vi "up_grid_data.vi"(9 "Data.V_Downstream":T1, 10 "Data.V_UpStream":T1) -> (0 "DOWN_Angle [Deg]":dbl, 1 "UP_Angle [Deg]":dbl, 2 "upper layer grid info":T3, 5 "DOWN_Angle_unwrap":dbl, 7 "UP_Angle_unwrap":dbl)   [LabVIEW 2021]
uses:
  3ph Phasor.ctl
  Phasor.ctl
  <vilib>/Analysis/coordinate.llb/Wrap Angle (scalar).vi
  <vilib>/Analysis/baseanly.llb/Complex A x Vector.vi
  <vilib>/Analysis/baseanly.llb/Mean (DBL).vi
  <vilib>/Analysis/Matrix/Numeric/Conversions/Array To Matrix - CA2.vi
  <vilib>/Analysis/NI_AALBase.lvlib
  <vilib>/Analysis/Matrix/NI_Matrix.lvlib
  <vilib>/Analysis/NI_AAL_Angle.lvlib
  <vilib>/Analysis/NI_AALPro.lvlib
panel:
  in  "y":dbl
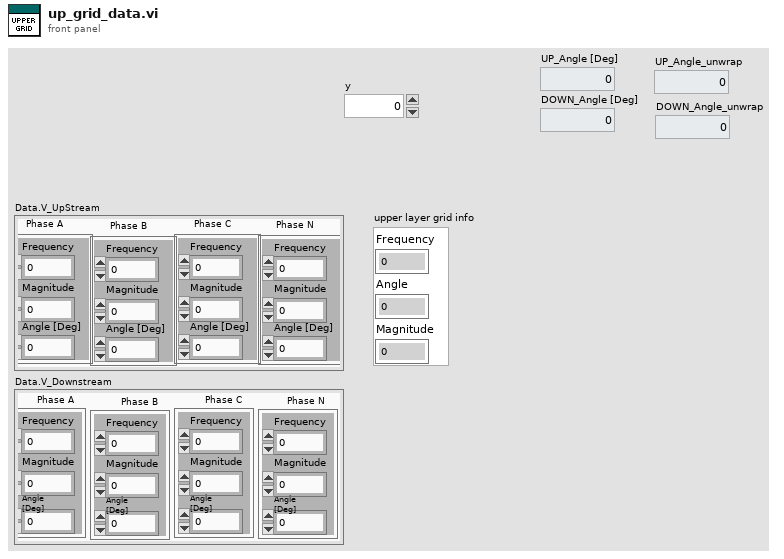
[diagram p1: front panel]
types:
  T1 = typedef "3ph Phasor.ctl" = cluster{"Phase A":T2, "Phase B":T2, "Phase C":T2, "Phase N":T2}
  T2 = typedef "Phasor.ctl" = cluster{"Frequency":dbl, "Magnitude":dbl, "Angle [Deg]":dbl}
  T3 = cluster{"Frequency":dbl, "Angle":dbl, "Magnitude":dbl}
  T4 = typedef "NI_Matrix.lvlib/ComplexMatrix.ctl" = cdb[][]
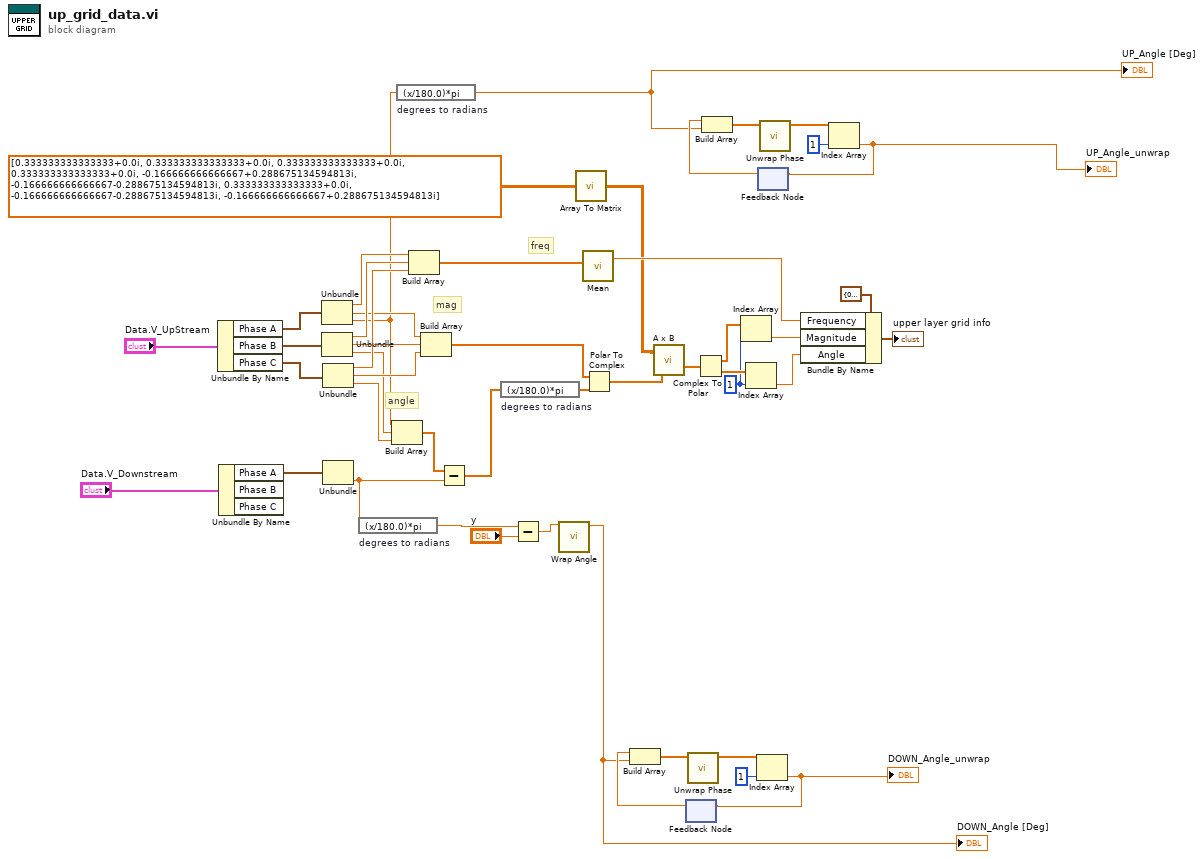
[diagram p0: block diagram]
diagram:
  w27 = 1 ("index")
  # "angle"
  # "mag"
  # "freq"
  n1 = Unbundle By Name("Data.V_UpStream") -> ("Phase A"=w45:T2, "Phase B"=w44:T2, "Phase C"=w43:T2)
  n2 = Unbundle By Name("Data.V_Downstream") -> ("Phase A"=w26:T2)  [unwired: 2 out]
  n3 = Unbundle(w45) -> ("Frequency"=w42:dbl, "Magnitude"=w39:dbl, "Angle [Deg]"=w17:dbl)
  n4 = Unbundle(w44) -> ("Frequency"=w41:dbl, "Magnitude"=w38:dbl, "Angle [Deg]"=w36:dbl)
  n5 = Unbundle(w43) -> ("Frequency"=w40:dbl, "Magnitude"=w37:dbl, "Angle [Deg]"=w35:dbl)
  n6 = Unbundle(w26) -> ("Angle [Deg]"=w16:dbl)  [unwired: 2 out]
  n7 = expression code="(x/180.0)*pi" "degrees to radians"(w16) -> (w2:dbl)
  n8 = Build Array(w17, w36, w35) -> (w18:dbl[])
  n9 = expression code="(x/180.0)*pi" "degrees to radians"(w17) -> (w3:dbl)
  "UP_Angle [Deg]" <- w3
  n10 = Build Array(w42, w41, w40) -> (w33:dbl[])
  n11 = Build Array(w39, w38, w37) -> (w32:dbl[])
  n12 = Subtract(x=w18, y=w16) -> (x-y=w19:dbl[])
  n13 = expression code="(x/180.0)*pi" "degrees to radians"(w19) -> (w20:dbl[])
  n14 = Subtract(x=w2, y="y") -> (x-y=w14:dbl)
  n15 = call-poly <vilib>:"Wrap Angle.vi"("angle in"=w14) -> ("angle out"=w1:dbl)  [unwired: 9 in, 1 out]
  "DOWN_Angle [Deg]" <- w1
  n16 = call-poly <vilib>:"Array To Matrix.vi"("Complex 2D Array"=cdb[][] [[0.333333333333333+0.0i, 0.333333333333333+0.0i, 0.333333333333333+0.0i], [0.333333333333333+0.0i, -0.166666666666667+0.288675134594813i, -0.166666666666667-0.288675134594813i], [0.333333333333333+0.0i, -0.166666666666667-0.288675134594813i, -0.166666666666667+0.288675134594813i]] ("r * e^(i*theta)")) -> ("Complex Matrix"=w21:T4)
  n17 = call-poly <vilib>:"Mean.vi"("X"=w33) -> ("mean"=w34:dbl)  [unwired: 1 out]
  n18 = Polar To Complex(1:w20, 2:w32) -> (0:w24:cdb[])
  n19 = call-poly <vilib>:"A x B.vi"("Vector"=w24, "A"=w21) -> ("A x Vector"=w23:cdb[])  [unwired: 1 out]
  n20 = feedback #1() -> (w6:dbl)  [unwired: 1 in]
  n21 = Build Array(w6, w1) -> (w12:dbl[])
  n22 = call <vilib>:"Unwrap Phase.vi"("Phase"=w12) -> ("Unwrapped Phase"=w13:dbl[])  [unwired: 9 in, 1 out]
  n23 = Complex To Polar ("Complex To Polar.vi")(r * e^(i*theta)=w23) -> (r=w30:dbl[], theta=w28:dbl[])
  n24 = Index Array(array=w30, index=w27) -> (element=w31:dbl)
  n25 = Index Array(array=w28, index=w27) -> (element=w29:dbl)
  n26 = Index Array(array=w13, index=1) -> (element=w5:dbl)
  "DOWN_Angle_unwrap" <- w5
  n27 = feedback-in #1(w5) -> ()
  n28 = feedback #2() -> (w8:dbl)  [unwired: 1 in]
  n29 = Build Array(w8, w3) -> (w9:dbl[])
  n30 = call <vilib>:"Unwrap Phase.vi"("Phase"=w9) -> ("Unwrapped Phase"=w10:dbl[])  [unwired: 9 in, 1 out]
  n31 = Bundle By Name(cluster=T3 {"Frequency"=0.0, "Angle"=0.0, "Magnitude"=0.0} ("upper layer grid info"), "Frequency"=w34, "Magnitude"=w31, "Angle"=w29) -> (→"upper layer grid info":T3)
  n32 = Index Array(array=w10, index=1) -> (element=w4:dbl)
  "UP_Angle_unwrap" <- w4
  n33 = feedback-in #2(w4) -> ()
